vi "GetText.vi"(8 "error in":errorcluster, 11 "TDMS datalogger editor node in":refnum<class "TDMS datalogger editor node.lvclass">) -> (0 "error out":errorcluster, 1 "additional text":string, 2 "text":string, 3 "TDMS datalogger editor node out":refnum<class "TDMS datalogger editor node.lvclass">, 4 "glyph":string)   [LabVIEW 2013, in "TDMS datalogger editor node.lvclass"]
uses:
  TDMS datalogger editor node.lvclass
  <vilib>/NI/Tag Bus Data Framework/Configuration Editor/Classes/Module editor node/Read display name.vi
  <vilib>/NI/Tag Bus Data Framework/Configuration Editor/PL Framework Configuration Tool.lvlib
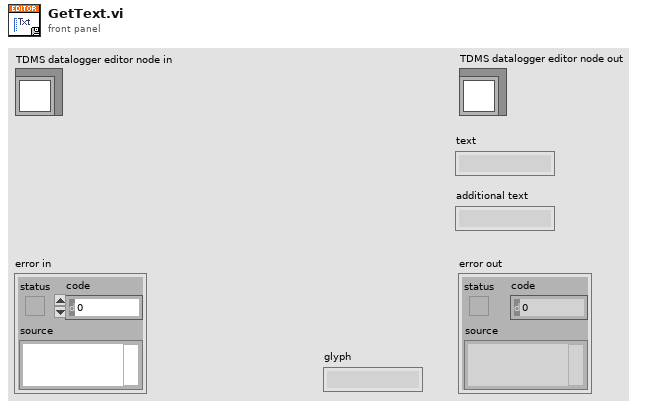
[diagram p1: front panel]
types:
  T1 = typedef "PL Framework Configuration Tool.lvlib/Glyphs Status.ctl" = enum16{"Normal", "Error", "Async"}
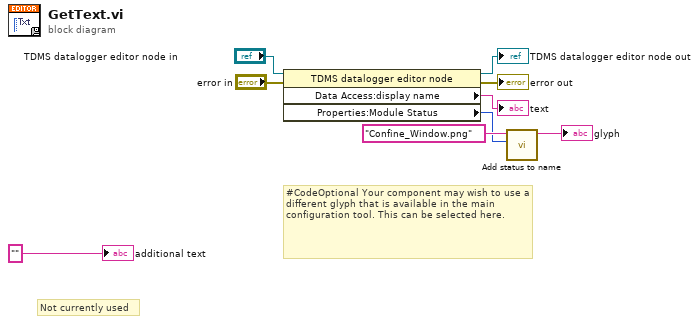
[diagram p0: block diagram]
diagram:
  # "Not currently used"
  # "#CodeOptional Your component may wish to use a different glyph that is available in the main configuration tool. This can be selected here."
  n1 = property class="TDMS datalogger editor node"(reference="TDMS datalogger editor node in", error in="error in") -> (reference out=→"TDMS datalogger editor node out":refnum<class "TDMS datalogger editor node.lvclass">, error out=→"error out":errorcluster, "Data Access:display name"=→"text":string, "Properties:Module Status"=w8:T1)
  n2 = call <vilib>:"Add status to name.vi"("Status"=w8, "Name"="Confine_Window.png" ("glyph")) -> ("Name with status"=→"glyph":string)  [unwired: 9 in]
  "additional text" <- "" ("additional text")
